vi "Dashboard Main.vi"() -> ()   [LabVIEW 2019]
uses:
  <vilib>/Utility/miscctls.llb/LVRowAndColumnTypeDef.ctl
  <vilib>/event_ctls.llb/eventvkey.ctl
  <vilib>/Rock Robotics/Network Tables/NT Read Numeric Array.vi
  <vilib>/Rock Robotics/WPI/Dashboard/WPI_DashboardLogging Global.vi
  <vilib>/Rock Robotics/Network Tables/NT Read Boolean.vi
panel:
  in  "Camera Settings Right":T1={"Frame Rate"=30, "Compression"=30, "Size"=1, "DB Camera Config"=FALSE} {"Frame Rate" scale=1.0..30.0; "Compression" scale=100.0..-1.0; "Size" items=["640x480", "320x240", "160x120"]}
  in  "Camera Name Right":string(combo)="No Camera Selection"
  out "Camera Perf":string
  in  "Camera Settings":T1={"Frame Rate"=30, "Compression"=30, "Size"=1, "DB Camera Config"=FALSE} {"Frame Rate" scale=1.0..30.0; "Compression" scale=100.0..-1.0; "Size" items=["640x480", "320x240", "160x120"]}
  in  "TCP":refnum<k5>
  in  "Rec Mode":enum32{"Stop", "Record", "Playback"}(radio)
  out "Robot IP":string
  out "Image Message":string="Timeout in Camera Communications"
  in  "Dashboard Tab":T2(tab)
  in  "Select Auto":string(combo)="Select Autonomous ..."
  out "NT Connection":bool
  out "MotorChart R":cluster{"Numeric":dbl, "Numeric":dbl}(graph)
  out "MotorChart L":cluster{"Numeric":dbl, "Numeric":dbl}(graph)
  out "MotorSliders R":cluster{"MotorSlide1":dbl, "MotorSlide2":dbl} {"MotorSlide2" scale=-1.0..1.0 scale format="%#_2e"; "MotorSlide1" scale=-1.0..1.0 scale format="%#_2e"}
  out "MotorSliders L":cluster{"MotorSlide1":dbl, "MotorSlide2":dbl} {"MotorSlide2" scale=-1.0..1.0 scale format="%#_2e"; "MotorSlide1" scale=-1.0..1.0 scale format="%#_2e"}
  out "Gyro":dbl(knob) scale=0.0..360.0
  out "JS1 Z":dbl(slide) scale=-1.0..1.0 scale format="%#_2e"
  out "JS1 Graph":cluster{"X":dbl, "Y":dbl}[](graph)
  out "JS1 Buttons":T3
  out "JS2 Z":dbl(slide) scale=-1.0..1.0 scale format="%#_2e"
  out "JS2 Graph":cluster{"X":dbl, "Y":dbl}[](graph)
  out "JS2 Buttons":T3
  out "Mode":T4(ring)=enum."Auto Disabled"
  out "Right Camera Perf":cluster{"Bandwidth (Mbps)":dbl, "FPS":dbl}
  out "x":sgl
  out "y":sgl
  out "Camera Image Right":T5(plugin-control)
  in  "DB/String 9":string
  in  "DB/String 8":string
  in  "DB/String 7":string
  in  "DB/String 6":string
  in  "DB/String 5":string
  in  "DB/String 4":string
  in  "DB/String 3":string
  in  "DB/String 2":string
  in  "DB/String 1":string
  in  "DB/String 0":string
  in  "DB/Slider 0":dbl(slide) scale=0.0..5.0
  in  "DB/Slider 1":dbl(slide) scale=0.0..5.0
  in  "DB/Slider 2":dbl(slide) scale=0.0..5.0
  in  "DB/Slider 3":dbl(slide) scale=0.0..5.0
  out "DB/LED 3":bool
  out "DB/LED 2":bool
  out "DB/LED 1":bool
  out "DB/LED 0":bool
  in  "DB/Button 3":bool
  in  "DB/Button 2":bool
  in  "DB/Button 1":bool
  in  "DB/Button 0":bool caption="New Name"
  in  "Test Slider":dbl(slide) scale=0.0..100.0 scale format="%#_3g"
  in  "On/Off":bool caption="Solenoid"
  in  "Test Name":u16(ring) items=["Select the test to run..."]
  in  "Test Tree":string(tree)
  in  "Motor":cluster{"Value":dbl, "Enable":bool} {"Value" scale=-1.0..1.0 scale format="%#_3g"}
  out "Progress":T6 {"Test Progress" scale=0.0..100.0}
  in  "Rev/Fwd":cluster{"Forward":bool, "Reverse":bool}
  in  "Test Ring":u16(ring) items=["Monochrome", "Color"]
  out "Cmd Status":string
  in  "Execute Command":bool
  in  "Command Params":string[][](table)
  in  "Command Selection":i32(listbox)
  in  "CheckList":i32(listbox)
  out "Tree":string(tree)
  out "Camera Image":T5(plugin-control)
  out "Background":bool
  in  "Camera Name":string(combo)="No Camera Selection"
  # "HW"
  # "HW"
  # "Joysticks"
  # "Drive Motors"
  # "Front"
  # "Right"
  # "Left"
  # "Back"
  # "This tab is a great place for autonomous settings and robot-specific values.\nPlace controls and indicators inside this tab and match name to\nDashboard Variables on robot. You can also delete this comment."
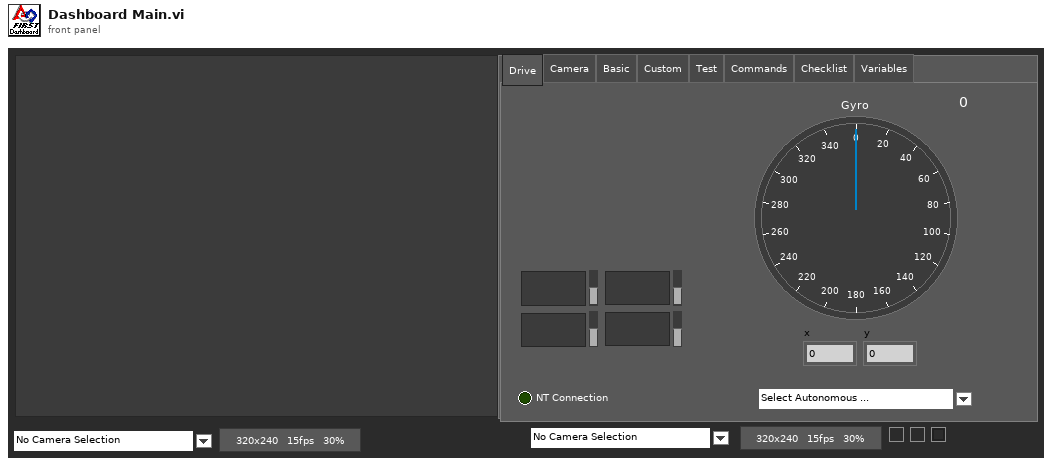
[diagram p1: front panel]
types:
  T1 = cluster{"Frame Rate":i32, "Compression":i32, "Size":u16, "DB Camera Config":bool}
  T2 = enum32{"Drive", "Camera", "Basic", "Custom", "Test", "Commands", "Checklist", "Variables"}
  T3 = cluster{bool, bool, bool, bool, bool, bool, bool, bool, bool, bool, bool, bool}
  T4 = enum8{"Tele-Op Disabled", "Tele-Op Enabled", "Auto Disabled", "Auto Enabled", "Test Disabled", "Test Enabled", "Disconnected", "No Code", "E-Stop"}
  T5 = typedef "IMAQ Image.ctl" = refnum<image>
  T6 = cluster{"Test Progress":u8, "Test Progress Text":string}
  T7 = cluster{"Save Path":path, "Interval (s)":dbl, "Keep":i32}
  T8 = typedef "Image Type" = u32
  T9 = cluster{"IDs":cluster{"RPC field ID":u16, "Unique ID":u16}, "String":string}
  T10 = cluster{"Camera Image":refnum<vi>, "Dashboard Tab":refnum<vi>, "Background":refnum<vi>, "Rec Mode":refnum<vi>, "Test Slider":refnum<vi>, "On/Off ":refnum<vi>, "Test Ring":refnum<vi>, "Rev/Fwd":refnum<vi>, "Test Name":refnum<vi>, "Motor":refnum<vi>, "Progress":refnum<vi>, "CheckList":refnum<vi>, "Tree":refnum<vi>, "Test Tree":refnum<vi>, "Command Params":refnum<vi>, "Command Selection":refnum<vi>, "Execute Command":refnum<vi>, "Cmd Status":refnum<vi>, "Camera Settings":refnum<vi>, "Camera Name":refnum<vi>, "Camera Perf":refnum<vi>, "Camera Settings Right":refnum<vi>, "Camera Name Right":refnum<vi>, "Camera Image Right":refnum<vi>}
  T11 = cluster{"Global Rectangle":i32[], "Contours":cluster{"Contour Type":u32, "ROI Type":u32, "Points":i32[]}[]}
  T12 = cluster{"Camera Name Right":string, string, "Saved DB Images Info":cluster{"Save Path":path, "Interval (s)":dbl, "Keep":i32}}
  T13 = cluster{"Error Strings":string, "Disable Counts":cluster{u16, u16}, "Rail Faults":cluster{u16, u16, u16}, "Robot IP":string, "DB Mode":u8, "Event Info":cluster{"Name":string, "Type":u8, "Number":u16, "Replay":u8}}
  T14 = cluster{"Storage":cluster{"Disk Free":u64, "RAM Block":u32, "RAM free":u32}, "CPU Utilization":cluster{"CPU % ISR":sgl, "CPU % Time Crit":sgl, "CPU % Timed Str":sgl, "CPU % High":sgl, "CPU % Above":sgl, "CPU % Normal":sgl, "CPU % Low":sgl}, "CAN":cluster{"% Bus Utilization":sgl, "Bus Off Cnt":u32, "TX_FIFO Full Cnt":u32, "Receive Error Cnt":u8, "Transmit Error Cnt":u8}, "HID":cluster{"HID Outputs":u32, "Rumble Low":u16, "Rumble High":u16}[]}
  T15 = cluster{"Status bits":cluster{"Test Mode":bool, "Autonomous":bool, "Enabled":bool, "Code Start":bool, "Brownout":bool, "Reserved 2":bool, "Reserved 3":bool, "E-Stop":bool}, "Code Trace":cluster{"Disabled":bool, "TeleOp":bool, "Auto":bool, "Test":bool}, "Controller Type":enum16{"unknown", "cRIO", "roboRio"}, "Code?":enum16{"unknown", "noCode", "code"}, "Battery V":dbl}
  T16 = cluster{"Control Bits":cluster{"TestMode":bool, "Autonomous":bool, "Enabled":bool, "FMS Present":bool, bool, bool, bool, "E-Stop":bool}, "Team Station ":u8, "Countdown":sgl, "Joystick Values":cluster{"Axes":dbl[], "Buttons":bool[], "POVs":i16[]}[]}
  T17 = cluster{"Axes":dbl[], "Buttons":bool[], "POVs":i16[]}[]
  T18 = cluster{"Axes":dbl[], "Buttons":bool[], "POVs":i16[]}
  T19 = cluster{"Buttons[0]":bool, "Buttons[1]":bool, "Buttons[2]":bool, "Buttons[3]":bool, "Buttons[4]":bool, "Buttons[5]":bool, "Buttons[6]":bool, "Buttons[7]":bool, "Buttons[8]":bool, "Buttons[9]":bool, "Buttons[10]":bool, "Buttons[11]":bool}
  T20 = cluster{"Camera Name":string, string, "Saved DB Images Info":cluster{"Save Path":path, "Interval (s)":dbl, "Keep":i32}}
  T21 = cluster{"Position":cluster{"x":sgl, "y":sgl}, "Angle":sgl, "Scale":sgl, "Score":sgl, "Bounding Box":cluster{"x":sgl, "y":sgl}[]}[]
  T22 = cluster{"Position":cluster{"x":sgl, "y":sgl}, "Angle":sgl, "Scale":sgl, "Score":sgl, "Bounding Box":cluster{"x":sgl, "y":sgl}[]}
  T23 = cluster{"Operation":enum16{"Update", "Clear"}, "Color Box":u32}[]
  T24 = typedef "eventvkey.ctl" = enum16{"ASCII", "Enter", "Return", "Shift", "Ctrl", "Alt", "Cmd", "Opt", "Caps", "NumLock", "Clear", "Break", "Up", "Down", "Left", "Right", "Insert", "Delete", "Home", "End", "PageUp", "PageDown", "Escape", "Help", "Pause", "ScrollLock", "F1", "F2", "F3", "F4", "F5", "F6", "F7", "F8", "F9", "F10", "F11", "F12", "F13", "F14", "F15", "F16", "F17", "F18", "F19", "F20", "F21", "F22", "F23", "F24", "Play", "VolumeUp", "VolumeDown", "Mute", "Two Byte Char"}
  T25 = cluster{"Image Size":bool, "Image Type":bool, "Pixel Value":bool, "ROI Information":bool, "Zoom Factor":bool}
  T26 = cluster{"Operation":enum16{"Update", "Clear"}, "Color Box":u32}
  T27 = typedef "LVRowAndColumnTypeDef.ctl" = cluster{"Row":i32, "Column":i32}
  T28 = cluster{"Shift":bool, "Ctrl":bool, "Alt":bool, "Cmd":bool, "Opt":bool}
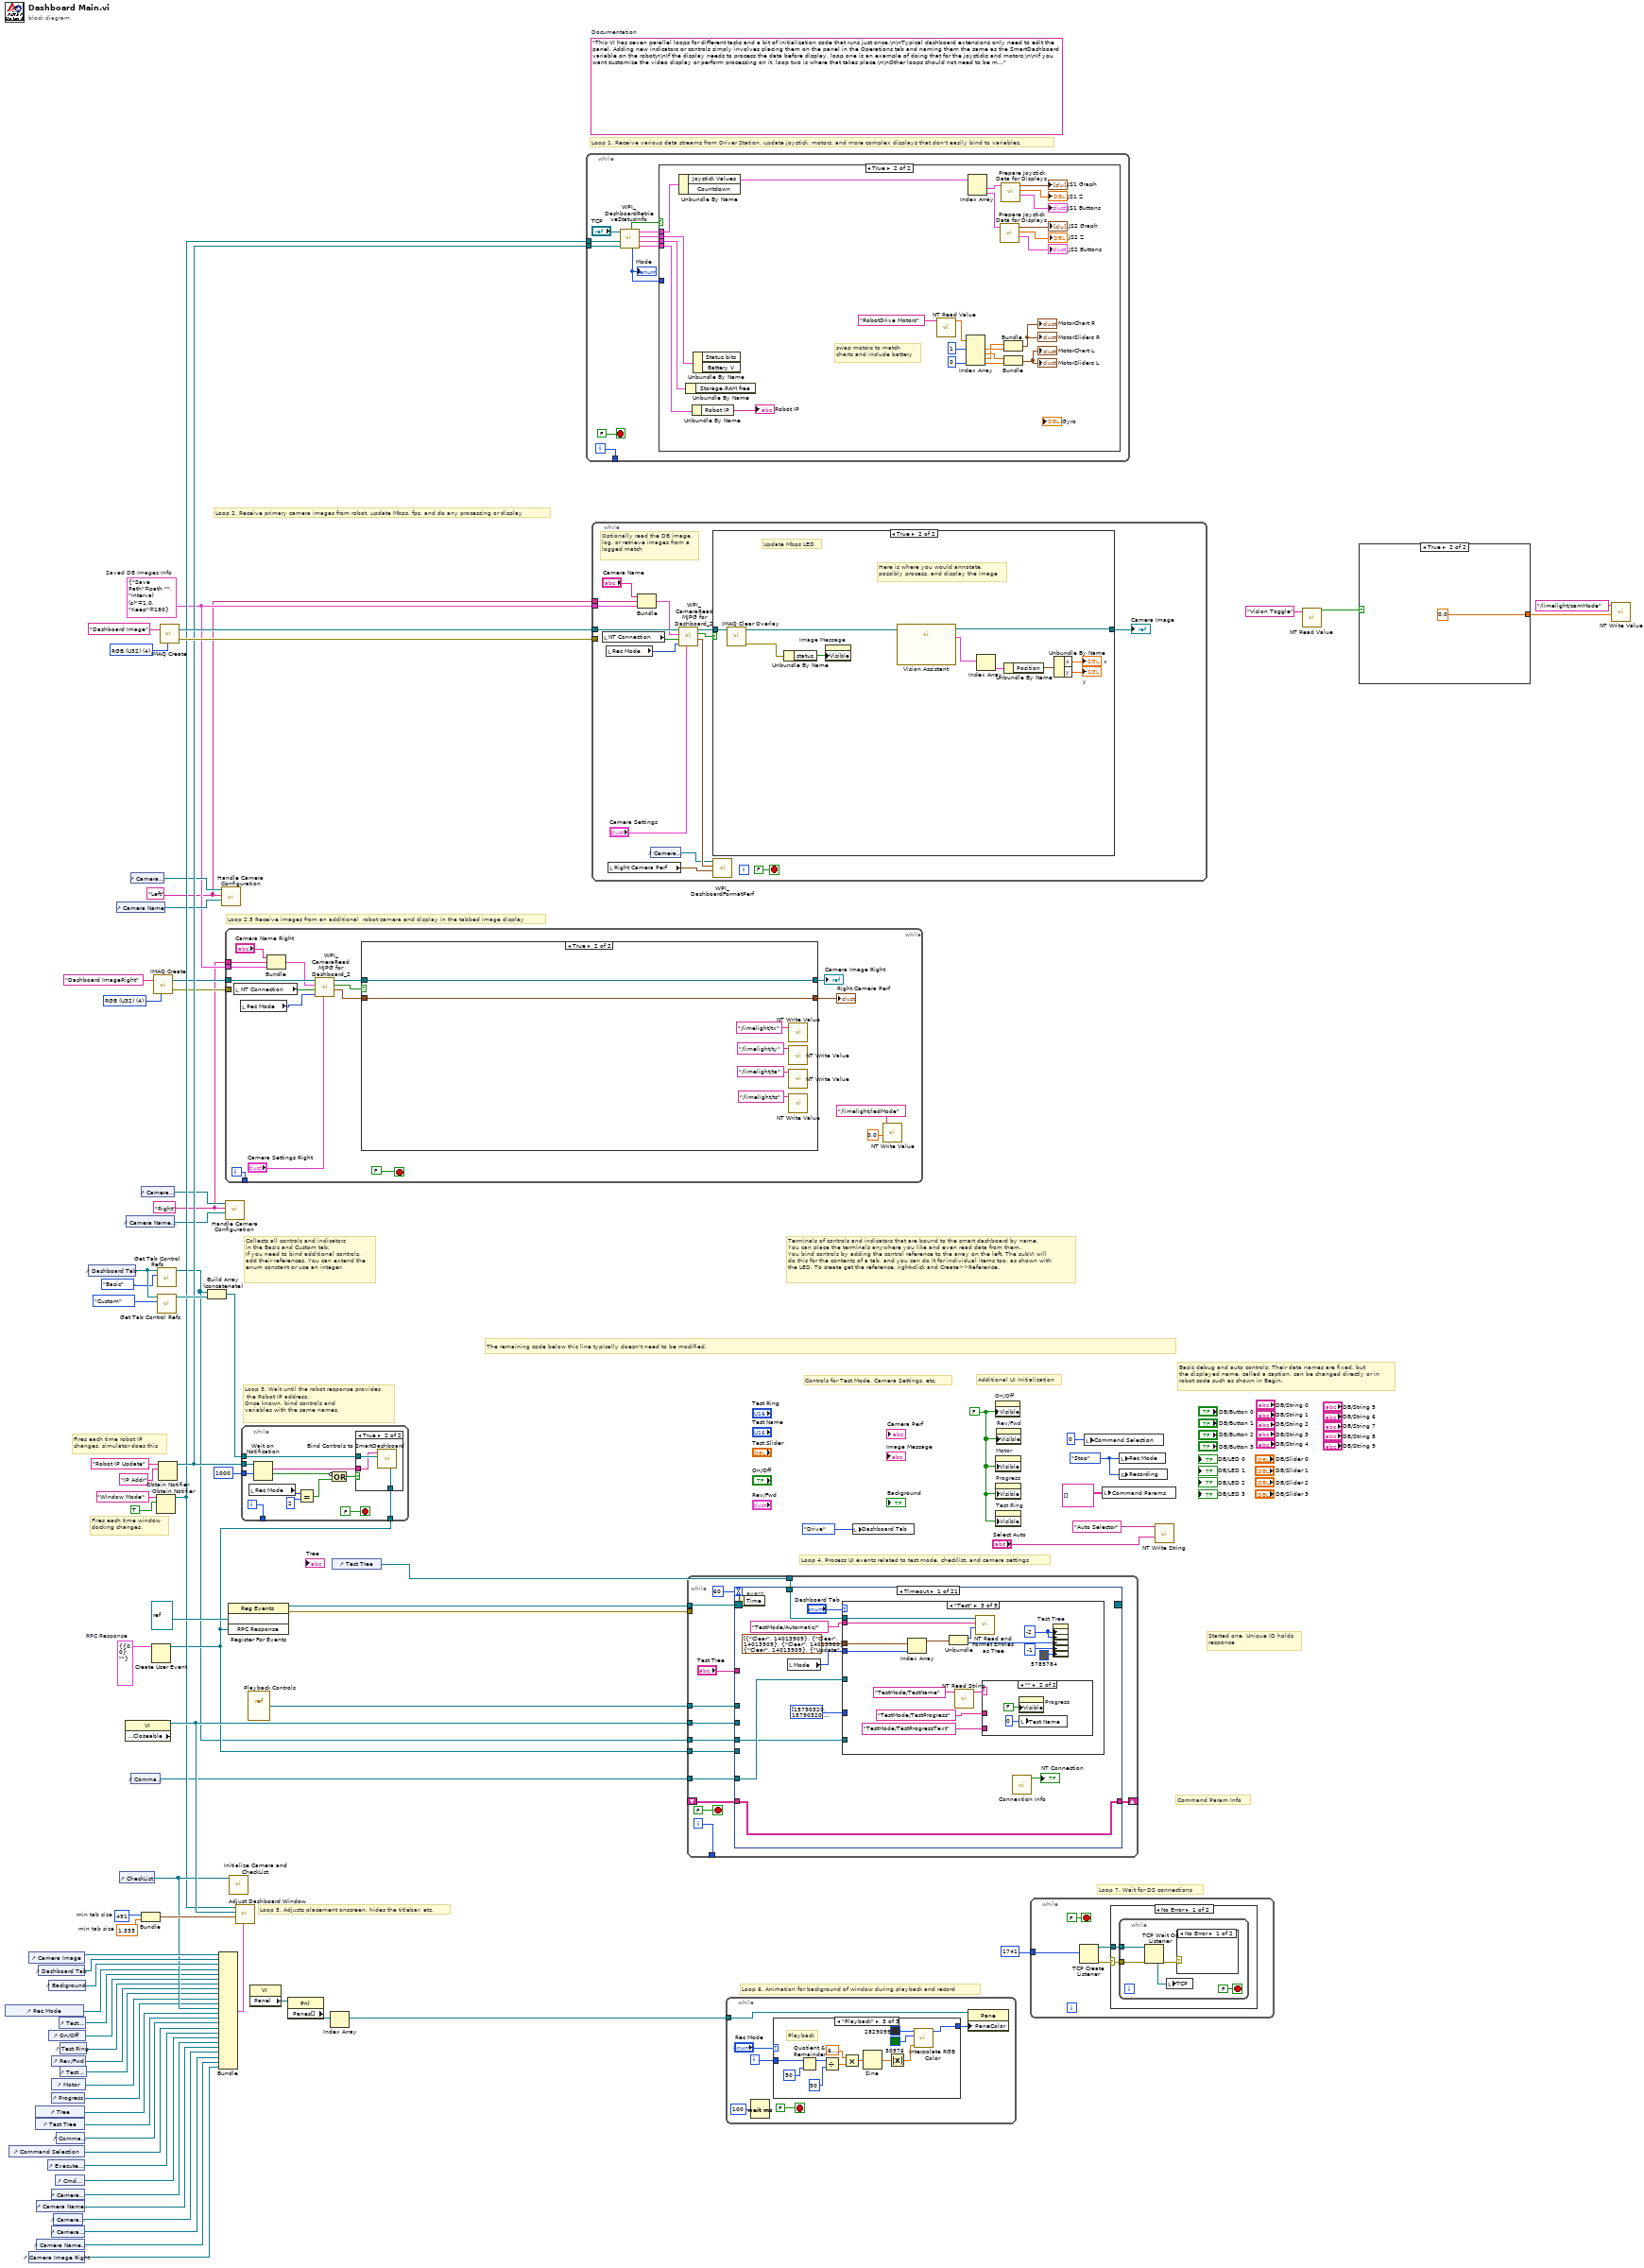
[diagram p0: block diagram]
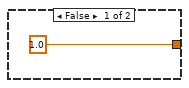
[diagram p2: hidden frame]
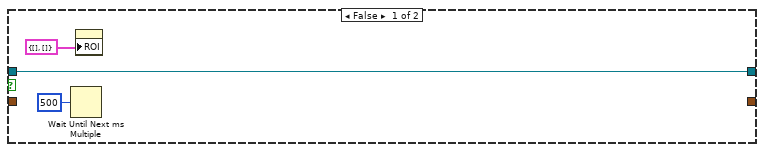
[diagram p3: hidden frame]
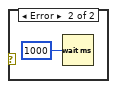
[diagram p4: hidden frame]
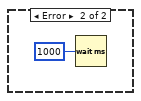
[diagram p5: hidden frame]
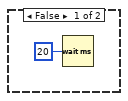
[diagram p6: hidden frame]
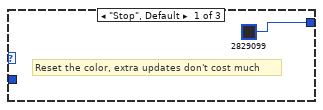
[diagram p7: hidden frame]
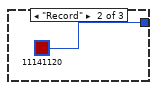
[diagram p8: hidden frame]
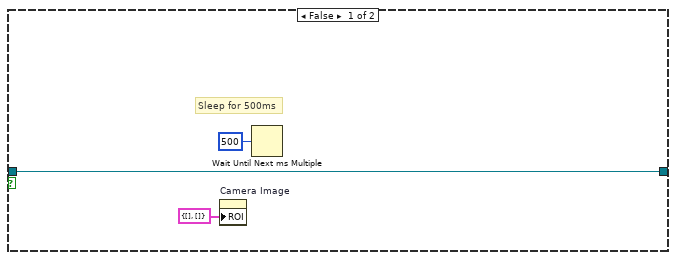
[diagram p10: hidden frame]
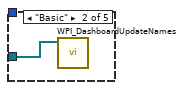
[diagram p12: hidden frame]
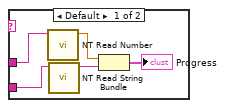
[diagram p13: hidden frame]
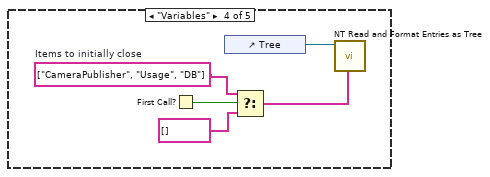
[diagram p14: hidden frame]
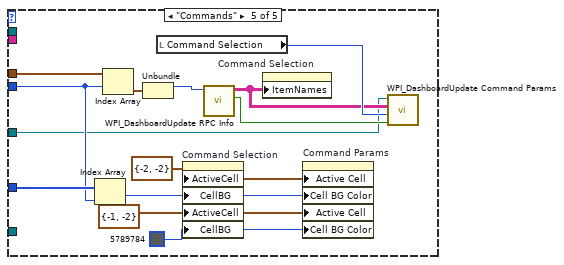
[diagram p15: hidden frame]
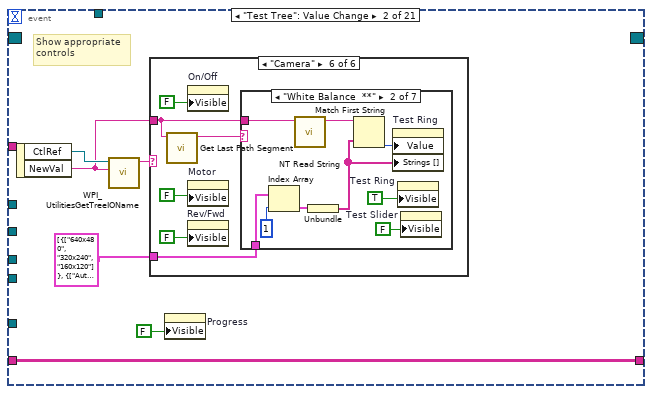
[diagram p16: hidden frame]
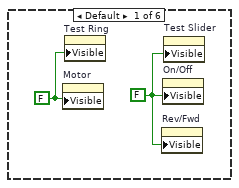
[diagram p17: hidden frame]
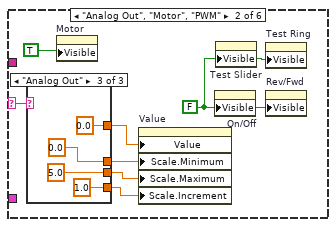
[diagram p18: hidden frame]
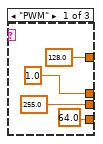
[diagram p19: hidden frame]
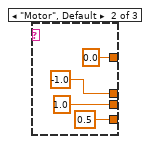
[diagram p20: hidden frame]
diagram:
  w7 = T7 {"Save Path"=path "", "Interval (s)"=1.0, "Keep"=180}  # Saved DB Images Info
  w6 = "Right"
  w5 = "Left"
  w17 = T8 4 items=["Grayscale (U8)", "Grayscale (I16)", "Grayscale (SGL)", "Complex (CSG)", "RGB (U32)", "HSL (U32)", "RGB (U64)"] ("Image Type")
  w33 = T9 {"IDs"={"RPC field ID"=0, "Unique ID"=0}, "String"=""}  # RPC Response
  w56 = 491  # min tab size
  w55 = 1.333  # min tab size
  w63 = enum32{"Stop", "Record", "Playback"}."Stop" ("Rec Mode")
  w40 = FALSE ("Visible")
  (unwired) "This VI has seven parallel loops for different tasks and a bit of initialization code that runs just once.\n\nTypical dashboard extensions only need to edit the panel. Adding new indicators or controls simply involves placing them on the panel in the Operations tab and naming them the same as the SmartDashboard variable on the robot\n\nIf the display needs to process the data before display, loop one is an example of doing that for the joysticks and motors.\n\nIf you want customize the video display or perform processing on it, loop two is where that takes place.\n\nOther loops should not need to be modified. They are pretty standard, and document the task they perform."  # Documentation
  w80 = T8 4 items=["Grayscale (U8)", "Grayscale (I16)", "Grayscale (SGL)", "Complex (CSG)", "RGB (U32)", "HSL (U32)", "RGB (U64)"] ("Image Type")
  # "Loop 2.5 Receive images from an additional  robot camera and display in the tabbed image display"
  # "Command Param Info"
  # "Started one, Unique ID holds\nresponse"
  # "Loop 7. Wait for DS connections"
  # "Basic debug and auto controls: Their data names are fixed, but\nthe displayed name, called a caption, can be changed directly or in\nrobot code such as shown in Begin."
  # "Controls for Test Mode, Camera Settings, etc."
  # "Additional UI Initialization"
  # "Loop 6. Animation for background of window during playback and record"
  # "Fires each time robot IP\nchanges, simulator does this"
  # "Fires each time window\ndocking changes."
  # "Collects all controls and indicators\nin the Basic and Custom tab.\nIf you need to bind additional controls,\nadd their references. You can extend the\nenum constant or use an integer."
  # "The remaining code below this line typically doesn't need to be modified."
  # "Loop 4. Process UI events related to test mode, checklist, and camera settings"
  # "Terminals of controls and indicators that are bound to the smart dashboard by name.\nYou can place the terminals anywhere you like and even read data from them.\nYou bind controls by adding the control reference to the array on the left. The subVI will\ndo this for the contents of a tab, and you can do it for individual items too, as shown with\nthe LED. To create get the reference, right-click and Create>>Reference."
  # "Loop 3. Wait until the robot response provides\n the Robot IP address.\nOnce known, bind controls and\nvariables with the same names."
  # "Loop 5. Adjusts placement onscreen, hides the titlebar, etc."
  # "Loop 1. Receive various data streams from Driver Station, update joystick, motors, and more complex displays that don't easily bind to variables."
  # "Loop 2. Receive primary camera images from robot, update Mbps, fps, and do any processing or display"
  n1 = control-ref of="Rec Mode"() -> (w46:refnum<vi>)
  n2 = control-ref of="Command Selection"() -> (w32:refnum<vi>)
  n3 = control-ref of="Camera Image Right"() -> (w10:refnum<vi>)
  n4 = control-ref of="Camera Image"() -> (w58:refnum<vi>)
  n5 = control-ref of="Tree"() -> (w50:refnum<vi>)
  n6 = control-ref of="Test Tree"() -> (w49:refnum<vi>)
  n7 = control-ref of="Camera Name"() -> (w23:refnum<vi>)
  n8 = control-ref of="Camera Name Right"() -> (w11:refnum<vi>)
  n9 = control-ref of="Dashboard Tab"() -> (w57:refnum<vi>)
  n10 = control-ref of="Execute Command"() -> (w34:refnum<vi>)
  n11 = control-ref of="Background"() -> (w53:refnum<vi>)
  n12 = control-ref of="On/Off"() -> (w44:refnum<vi>)
  n13 = control-ref of="Progress"() -> (w41:refnum<vi>)
  n14 = control-ref of="Camera Settings"() -> (w24:refnum<vi>)
  n15 = control-ref of="Camera Settings Right"() -> (w12:refnum<vi>)
  n16 = control-ref of="Rev/Fwd"() -> (w42:refnum<vi>)
  n17 = control-ref of="Motor"() -> (w47:refnum<vi>)
  n18 = control-ref of="Camera Perf"() -> (w22:refnum<vi>)
  n19 = control-ref of="Cmd Status"() -> (w28:refnum<vi>)
  n20 = control-ref of="Command Params"() -> (w35:refnum<vi>)
  n21 = control-ref of="Test Slider"() -> (w45:refnum<vi>)
  n22 = control-ref of="Test Ring"() -> (w43:refnum<vi>)
  n23 = control-ref of="Test Name"() -> (w48:refnum<vi>)
  n24 = control-ref of="Dashboard Tab"() -> (w61:refnum<vi>)
  n25 = control-ref of="Camera Name"() -> (w25:refnum<vi>)
  n26 = control-ref of="CheckList"() -> (w51:refnum<vi>)
  n27 = property class="VI" props=["Front Panel.Closeable"]() -> (reference out=w62:refnum<vi>)  [unwired: 2 in, 2 out]
  n28 = control-ref of="Camera Name Right"() -> (w13:refnum<vi>)
  n29 = control-ref of="Camera Settings"() -> (w26:refnum<vi>)
  n30 = control-ref of="Command Params"() -> (w27:refnum<vi>)
  n31 = control-ref of="Camera Settings Right"() -> (w14:refnum<vi>)
  n32 = Bundle("min tab size"=w56, "min tab size"=w55) -> (w54:cluster{"min tab size":i32, "min tab size":dbl})  [unwired: 1 in]
  n33 = Create User Event(user event datatype=w33) -> (user event=w29:refnum<user-event>)  [unwired: 1 in, 1 out]
  n34 = call "IMAQ Create"("Image Name"="Dashboard ImageRight", "Image Type"=w17) -> ("New Image"=w16:T5, "error out"=w15:errorcluster)  [unwired: 2 in, 1 out]
  n35 = Obtain Notifier(name (unnamed)="Window Mode", notification data type=TRUE) -> (notifier out=w38:refnum<notifier>)  [unwired: 2 in, 2 out]
  n36 = call <vilib>:"Get Tab Control Refs.vi"("Page Index"=T2."Basic" ("Dashboard Tab"), "TabControl in"=w61) -> ("ControlsOnPage"=w21:refnum<vi>[])  [unwired: 9 in]
  n37 = call <vilib>:"Get Tab Control Refs.vi"("Page Index"=T2."Custom" ("Dashboard Tab"), "TabControl in"=w61) -> ("ControlsOnPage"=w60:refnum<vi>[])  [unwired: 9 in]
  n38 = Obtain Notifier(name (unnamed)="Robot IP Update", notification data type="IP Addr" ("name (unnamed)")) -> (notifier out=w39:refnum<notifier>)  [unwired: 2 in, 2 out]
  n39 = call "IMAQ Create"("Image Name"="Dashboard Image", "Image Type"=w80) -> ("New Image"=w78:T5, "error out"=w77:errorcluster)  [unwired: 2 in, 1 out]
  n40 = Build Array (concatenate)(w21, w60) -> (w59:refnum<vi>[])
  n41 = Bundle("Camera Image"=w58, "Dashboard Tab"=w57, "Background"=w53, "Rec Mode"=w46, "Test Slider"=w45, "On/Off"=w44, "Test Ring"=w43, "Rev/Fwd"=w42, "Test Name"=w48, "Motor"=w47, "Progress"=w41, "CheckList"=w51, "Tree"=w50, "Test Tree"=w49, "Command Params"=w35, "Command Selection"=w32, "Execute Command"=w34, "Cmd Status"=w28, "Camera Settings"=w24, "Camera Name"=w23, "Camera Perf"=w22, "Camera Settings Right"=w12, "Camera Name Right"=w11, "Camera Image Right"=w10) -> (w52:T10)  [unwired: 1 in]
  n42 = call "Handle Camera Configuration.vi"("CameraNameRef"=w25, "Display Name"=w5, "ClusterRef"=w26) -> ()  [unwired: 9 in]
  n43 = call "Handle Camera Configuration.vi"("CameraNameRef"=w13, "Display Name"=w6, "ClusterRef"=w14) -> ()  [unwired: 9 in]
  n44 = while {
    tunnel: w16 -> [w97]
    tunnel: w15 -> [_]
    tunnel: [w92] -> _
    tunnel: w7 -> [w89]
    tunnel: w6 -> [w86]
    i -> [w92]
    stop <- FALSE stop-if-true
    n45 = local read "NT Connection"() -> (w90:bool)
    n46 = local read "Rec Mode"() -> (w96:enum32{"Stop", "Record", "Playback"})
    n47 = Bundle("Camera Name Right"="Camera Name Right", w86, "Saved DB Images Info"=w89) -> (w88:T12)  [unwired: 1 in]
    n48 = call <vilib>:"WPI_CameraRead MJPG for Dashboard_2.vi"("Camera Settings"="Camera Settings Right", "Rec Mode"=w96, "NT Connection"=w90, "Capture Info"=w88, "Image in"=w97) -> ("perf info"=w84:cluster{"Bandwidth (Mbps)":dbl, "fps":dbl}, "Active"=w91:bool, "Image\\ out"=w94:T5)  [unwired: 4 in]
    n49 = case shown="True" w91 {
      tunnel: w94 -> [w99 w101]
      tunnel: [w99 w101] -> w81
      tunnel: [_ w106] -> w85
      tunnel: w84 -> [_ w106]
      frame False {
        n50 = Wait Until Next ms Multiple(millisecond multiple=u32 500) -> ()  [unwired: 1 out]
        n51 = property on="Camera Image Right" class="ImageControl"("ROI"=T11 {"Global Rectangle"=[], "Contours"=[]}) -> ()  [unwired: 2 in, 2 out]
      }
      frame True {
        n52 = call-poly <vilib>:"NT Write Value.vi"("Name"="/limelight/tx") -> ()  [unwired: 10 in, 1 out]
        n53 = call-poly <vilib>:"NT Write Value.vi"("Name"="/limelight/ty") -> ()  [unwired: 10 in, 1 out]
        n54 = call-poly <vilib>:"NT Write Value.vi"("Name"="/limelight/ta") -> ()  [unwired: 10 in, 1 out]
        n55 = call-poly <vilib>:"NT Write Value.vi"("Name"="/limelight/ts") -> ()  [unwired: 10 in, 1 out]
      }
    }
    "Right Camera Perf" <- w85
    "Camera Image Right" <- w81
    n56 = call-poly <vilib>:"NT Write Value.vi"("Numeric"=0.0, "Name"="/limelight/ledMode") -> ()  [unwired: 9 in, 1 out]
  }
  n57 = register-events(refnum<vi> refnum, w29) -> (reference out=w67:refnum<event-registration>, error out=w66:errorcluster)  [unwired: 2 in]
  n58 = call "Initialize Camera and CheckList.vi"("ListBox in"=w51) -> ()  [unwired: 11 in]
  n59 = call "Adjust Dashboard Window.vi"("Sizing Refnums"=w52, "Size Constraints"=w54, "VI"=w62, "WIn Mode"=w38) -> ()  [unwired: 8 in]
  n60 = while {
    tunnel: w59 -> [w118]
    tunnel: w39 -> [w116]
    tunnel: [w114] -> _
    tunnel: u32 1000 ("milliseconds to wait") -> [w113]
    tunnel: w29 -> [w107]
    i -> [w114]
    stop <- FALSE stop-if-true
    n61 = local read "Rec Mode"() -> (w109:enum32{"Stop", "Record", "Playback"})
    n62 = Wait on Notification(notifier=w116, timeout in ms (-1)=w113) -> (notification=w115:string, timed out?=w111:bool)  [unwired: 2 in, 2 out]
    n63 = Equal?(x=w109, y=u16 2 ("Rec Mode")) -> (x = y?=w110:bool)
    n64 = Compound Arithmetic op=OR(invert w111, w110) -> (w112:bool)
    n65 = case shown="True" w112 {
      tunnel: w118 -> [_ w121]
      tunnel: w115 -> [_ w120]
      tunnel: w107 -> [_ w119]
      frame False {
      }
      frame True {
        n66 = call <vilib>:"Bind Controls to SmartDashboard.vi"("RPC ref"=w119, "Bound Control Refs"=w121, "Server IP Address"=w120) -> ()  [unwired: 9 in]
      }
    }
  }
  n67 = vi-ref "Playback Controls.vi"() -> (w68:refnum<vi>)
  n68 = property class="VI"() -> ("Panel"=w70:refnum<vi>)  [unwired: 2 in, 2 out]
  n69 = property class="Pnl"(reference=w70) -> ("Panes[]"=w71:refnum<vi>[])  [unwired: 1 in, 2 out]
  n70 = Index Array(array=w71) -> (element=w69:refnum<vi>)  [unwired: 1 in]
  n71 = control-ref of="Test Tree"() -> (w72:refnum<vi>)
  n72 = while {
    tunnel: [w131] -> _
    tunnel: w39 -> [w125]
    tunnel: w38 -> [w122]
    i -> [w131]
    stop <- FALSE stop-if-true
    n73 = call <vilib>:"WPI_DashboardRetrieveStatusInfo.vi"("Binding Refnum"=w125, "Window Mode Notifier"=w122, "TCP Cnx"="TCP") -> ("Power and Errors"=w126:T13, "Robot Metrics"=w129:T14, "Status Info"=w130:T15, "Control Info"=w127:T16, "Robot Mode"=w124:T4, "Process?"=w128:bool)  [unwired: 3 in]
    "Mode" <- w124
    n74 = case shown="True" w128 {
      tunnel: w130 -> [_ w157]
      tunnel: w129 -> [_ w156]
      tunnel: w127 -> [_ w155]
      tunnel: w126 -> [_ w154]
      tunnel: w124 -> [_ _]
      frame False {
        n75 = Wait (ms)(milliseconds to wait=u32 20) -> ()  [unwired: 1 out]
      }
      frame True {
        # "swap motors to match\ncharts and include battery"
        n76 = Unbundle By Name(w155) -> ("Joystick Values"=w145:T17)  [unwired: 1 out]
        n77 = Unbundle By Name(w156) -> ()  [unwired: 1 out]
        n78 = Unbundle By Name(w154) -> ("Robot IP"=→"Robot IP":string)
        n79 = Unbundle By Name(w157) -> ()  [unwired: 2 out]
        n80 = call-poly <vilib>:"NT Read Value.vi"("Name"="RobotDrive Motors") -> ("Numeric Array"=w135:dbl[])  [unwired: 9 in, 1 out]
        n81 = Index Array(array=w135, index #1=1, index #4=0) -> (element #1=w149:dbl, element #2=w150:dbl, element #3=w148:dbl, element #4=w153:dbl)  [unwired: 2 in]
        n82 = Index Array(array=w145) -> (element #1=w144:T18, element #2=w140:T18)  [unwired: 2 in]
        n83 = call "Prepare Joystick Data for Displays.vi"("Joystick Values"=w140) -> ("Buttons"=→"JS2 Buttons":T19, "Z Axis"=→"JS2 Z":dbl, "Cartesian Data"=→"JS2 Graph":cluster{"X axis":dbl, "X axis":dbl}[])  [unwired: 8 in]
        n84 = call "Prepare Joystick Data for Displays.vi"("Joystick Values"=w144) -> ("Buttons"=→"JS1 Buttons":T19, "Z Axis"=→"JS1 Z":dbl, "Cartesian Data"=→"JS1 Graph":cluster{"X axis":dbl, "X axis":dbl}[])  [unwired: 8 in]
        n85 = Bundle("Numeric"=w148, "Numeric"=w149) -> (→"MotorChart R" →"MotorSliders R":cluster{"Numeric":dbl, "Numeric":dbl})  [unwired: 1 in]
        n86 = Bundle("Numeric"=w150, "Numeric"=w153) -> (→"MotorChart L" →"MotorSliders L":cluster{"Numeric":dbl, "Numeric":dbl})  [unwired: 1 in]
      }
    }
  }
  n87 = while {
    tunnel: w78 -> [w171]
    tunnel: w77 -> [_]
    tunnel: w7 -> [w165]
    tunnel: w5 -> [w162]
    stop <- FALSE stop-if-true
    # "Optionally read the DB image,\nlog, or retrieve images from a\nlogged match"
    n88 = local read "NT Connection"() -> (w166:bool)
    n89 = local read "Rec Mode"() -> (w168:enum32{"Stop", "Record", "Playback"})
    n90 = local read "Right Camera Perf"() -> (w160:cluster{"Bandwidth (Mbps)":dbl, "FPS":dbl})
    n91 = Bundle("Camera Name"="Camera Name", w162, "Saved DB Images Info"=w165) -> (w164:T20)  [unwired: 1 in]
    n92 = control-ref of="Camera Perf"() -> (w159:refnum<vi>)
    n93 = call <vilib>:"WPI_CameraRead MJPG for Dashboard_2.vi"("Camera Settings"="Camera Settings", "Rec Mode"=w168, "NT Connection"=w166, "Capture Info"=w164, "Image in"=w171) -> ("perf info"=w161:cluster{"Bandwidth (Mbps)":dbl, "fps":dbl}, "Active"=w169:bool, "Image\\ out"=w170:T5)  [unwired: 4 in]
    n94 = case shown="True" w169 {
      tunnel: w170 -> [w174 w183]
      tunnel: [w174 w181] -> w158
      frame False {
        # "Sleep for 500ms"
        n95 = property on="Camera Image" class="ImageControl"("ROI"=T11 {"Global Rectangle"=[], "Contours"=[]}) -> ()  [unwired: 2 in, 2 out]
        n96 = Wait Until Next ms Multiple(millisecond multiple=u32 500) -> ()  [unwired: 1 out]
      }
      frame True {
        # "Here is where you would annotate,\npossibly process, and display the image"
        # "Update Mbps LED"
        n97 = call "IMAQ Clear Overlay"("Image"=w183) -> ("error out"=w184:errorcluster, "Image Out"=w182:T5)  [unwired: 2 in, 7 out]
        n98 = Unbundle By Name(w184) -> ("status"=w185:bool)
        n99 = property on="Image Message" class="Str"("Visible"=w185) -> ()  [unwired: 2 in, 2 out]
        n100 = call "Vision Assistant"("Image In"=w182) -> ("Image Out"=w181:T5, "Matches (Pattern Matching 1)"=w180:T21)  [unwired: 24 in, 1 out]
        n101 = Index Array(array=w180) -> (element=w179:T22)  [unwired: 1 in]
        n102 = Unbundle By Name(w179) -> ("Position"=w178:cluster{"x":sgl, "y":sgl})
        n103 = Unbundle By Name(w178) -> ("x"=→"x":sgl, "y"=→"y":sgl)
      }
    }
    "Camera Image" <- w158
    n104 = call <vilib>:"WPI_DashboardFormatPerf.vi"("Right Camera Perf"=w160, "Performance"=w161, "String in"=w159) -> ()  [unwired: 9 in]
  }
  n105 = while {
    tunnel: [w195] -> _
    tunnel: w72 -> [w194]
    tunnel: w68 -> [w193]
    tunnel: w67 -> [w192]
    tunnel: w66 -> [_]
    tunnel: w62 -> [w191]
    tunnel: w29 -> [w190]
    tunnel: w27 -> [w189]
    shift-right: [w188] -> _
    shift-left: _ -> [w187]
    tunnel: w21 -> [w186]
    i -> [w195]
    stop <- FALSE stop-if-true
    n106 = event shown="[0] Timeout" {
      selector: w192 -> [_ _ _ _ _ _ _ _ _ _ _ _ _ _ _ _ _ _ _ _ _]
      dyn-events: [_ _ _ _ _ _ _ _ _ _ _ _ _ _ _ _ w455 _ _ _ _] -> _
      timeout: u32 60 ("milliseconds to wait") -> [_ _ _ _ _ _ _ _ _ _ _ _ _ _ _ _ _ _ _ _ _]
      tunnel: w194 -> [w207 _ _ _ _ _ _ _ _ _ _ _ _ _ _ _ _ _ _ _ _]
      tunnel: "Test Tree" -> [_ _ _ _ _ _ _ _ _ _ _ w422 w430 w432 w436 w444 _ _ _ _ _]
      tunnel: w193 -> [_ _ _ _ _ _ _ _ _ _ _ _ _ _ _ _ w457 _ w475 _ _]
      tunnel: w191 -> [_ _ _ _ _ _ _ _ _ _ _ _ _ _ _ _ w453 _ _ _ _]
      tunnel: w190 -> [_ _ _ _ _ _ _ _ _ _ _ _ _ _ _ _ w451 _ _ _ _]
      tunnel: w189 -> [w202 _ _ _ _ _ w373 _ _ _ _ _ _ _ _ _ _ _ _ _ _]
      tunnel: [w201 w250 w352 w357 w366 w370 w371 w380 w390 w397 w409 w421 w428 w431 w435 w443 w450 w470 w472 w476 w489] -> w188
      tunnel: w187 -> [w201 w250 w352 w357 w366 w370 w371 _ _ w397 w409 w421 w428 w431 w435 w443 w450 w470 w472 w476 w489]
      tunnel: w186 -> [w199 _ _ _ _ _ _ _ _ _ _ _ _ _ _ _ _ _ _ _ _]
      event Timeout {
        n107 = event-data() -> ()  [unwired: 1 in, 1 out]
        n108 = local read "Mode"() -> (w204:T4)
        n109 = case shown="\"Test\"" "Dashboard Tab" {
          tunnel: w207 -> [_ _ w223 _ _]
          tunnel: "TestMode/Automatic/" ("Name Pattern") -> [_ _ w222 _ _]
          tunnel: T23 [{"Operation"=enum."Clear", "Color Box"=14013909}, {"Operation"=enum."Clear", "Color Box"=14013909}, {"Operation"=enum."Clear", "Color Box"=14013909}, {"Operation"=enum."Clear", "Color Box"=14013909}, {"Operation"=enum."Update", "Color Box"=14013909}, {"Operation"=enum."Update", "Color Box"=16777215}, {"Operation"=enum."Clear", "Color Box"=14013909}, {"Operation"=enum."Clear", "Color Box"=14013909}, {"Operation"=enum."Clear", "Color Box"=14013909}] -> [_ _ w215 _ w243]
          tunnel: w204 -> [_ _ w214 _ w242]
          tunnel: u32[] [15790320, 15790320, 15790320, 15790320, 16777215, 16777215, 15790320, 15790320, 15790320] -> [_ _ _ _ w248]
          tunnel: w202 -> [_ _ _ _ w236]
          tunnel: w199 -> [_ w209 _ _ _]
          frame "Custom", Default {
          }
          frame "Basic" {
            n110 = call <vilib>:"WPI_DashboardUpdateNames.vi"("Controls on Tab"=w209) -> ()  [unwired: 11 in]
          }
          frame "Test" {
            w221 = -2 ("Active Item:Row Number")
            n111 = Index Array(array=w215, index=w214) -> (element=w216:T26)
            n112 = Unbundle(w216) -> ("Operation"=w217:enum16{"Update", "Clear"}, "Color Box"=w218:u32)
            n113 = call <vilib>:"NT Read String.vi"("Name"="TestMode/TestName") -> ("String"=w212:string)  [unwired: 9 in, 1 out]
            n114 = call <vilib>:"NT Read and Format Entries as Tree.vi"("Operation"=w217, "Name Pattern"=w222, "Tree Refnum"=w223) -> ()  [unwired: 7 in, 2 out]
            n115 = case shown="\"\"" w212 {
              tunnel: "TestMode/TestProgress" ("Name") -> [w225 _]
              tunnel: "TestMode/TestProgressText" ("Name") -> [w224 _]
              frame Default {
                n116 = call <vilib>:"NT Read Number.vi"("Name"=w225) -> ("Numeric"=w226:dbl)  [unwired: 9 in, 1 out]
                n117 = call <vilib>:"NT Read String.vi"("Name"=w224) -> ("String"=w227:string)  [unwired: 9 in, 1 out]
                n118 = Bundle("Numeric"=w226, "String"=w227) -> (→"Progress":cluster{"Numeric":dbl, "String":string})  [unwired: 1 in]
              }
              frame "" {
                n119 = property on="Progress" class="Clust (strict)"("Visible"=FALSE) -> ()  [unwired: 2 in, 2 out]
                n120 = local write "Test Name"(u16 0) -> ()
              }
            }
            n121 = property on="Test Tree" class="Tree (strict)"("Active Item Row Number"=w221, "ActiveColNum"=w221, "CellBG"=w218, "Active Item Row Number"=-1 ("Active Item:Row Number"), "CellBG"=u32 5789784 ("Color Box")) -> ()  [unwired: 2 in, 2 out]
          }
          frame "Variables" {
            w233 = string[] ["CameraPublisher", "Usage", "DB"]  # Items to initially close
            n122 = First Call?() -> (First Call?: T/F=w234:bool)
            n123 = control-ref of="Tree"() -> (w235:refnum<vi>)
            n124 = Select(t=w233, s=w234, f=string[] []) -> (s? t:f=w231:string[])
            n125 = call <vilib>:"NT Read and Format Entries as Tree.vi"("Tags to  Close"=w231, "Tree Refnum"=w235) -> ()  [unwired: 8 in, 2 out]
          }
          frame "Commands" {
            w244 = u32 5789784 ("Color Box")
            w245 = T27 {"Row"=-1, "Column"=-2} ("Active Cell:Active Cell")
            w247 = T27 {"Row"=-2, "Column"=-2} ("Active Cell:Active Cell")
            n126 = Index Array(array=w248, index=w242) -> (element=w246:u32)
            n127 = Index Array(array=w243, index=w242) -> (element=w241:T26)
            n128 = Unbundle(w241) -> ("Operation"=w240:enum16{"Update", "Clear"})  [unwired: 1 out]
            n129 = local read "Command Selection"() -> (w239:i32)
            n130 = property on="Command Selection" class="MCListbox (strict)"("ActiveCell"=w247, "CellBG"=w246, "ActiveCell"=w245, "CellBG"=w244) -> ()  [unwired: 2 in, 2 out]
            n131 = call <vilib>:"WPI_DashboardUpdate RPC Info.vi"("Operation"=w240) -> ("update"=w238:bool, "commands"=w237:string[][])  [unwired: 9 in]
            n132 = property on="Command Selection" class="MCListbox (strict)"("ItemNames"=w237) -> ()  [unwired: 2 in, 2 out]
            n133 = property on="Command Params" class="Tbl (strict)"("Active Cell"=w247, "Cell BG Color"=w246, "Active Cell"=w245, "Cell BG Color"=w244) -> ()  [unwired: 2 in, 2 out]
            n134 = call <vilib>:"WPI_DashboardUpdate Command Params.vi"("Update"=w238, "NewVal"=w239, "Commands"=w237, "Param Tbl"=w236) -> ()  [unwired: 7 in, 1 out]
          }
        }
        n135 = call <vilib>:"Connextion Info.vi"() -> ("Connected"=→"NT Connection":bool)  [unwired: 10 in, 1 out]
      }
      event "Test Tree": Value Change {
        # "Show appropriate\ncontrols"
        n136 = event-data() -> ("CtlRef"=w253:refnum<vi>, "NewVal"=w251:string)  [unwired: 1 in]
        n137 = call <vilib>:"WPI_UtilitiesGetTreeIOName.vi"("NewVal"=w251, "TreeControl in"=w253) -> ("I/O Name"=w254:string)  [unwired: 9 in]
        n138 = case shown="\"Camera\"" w254 {
          selector: w254 -> [_ w261 _ w283 w292 _]
          tunnel: w251 -> [_ _ w280 w282 _ w299]
          tunnel: cluster{string[]}[] [{["640x480", "320x240", "160x120"]}, {["Auto", "Fixed indoor", "Fixed outdoor 1", "Fixed outdoor 2", "Fixed fluorescent 1", "Fixed fluorescent 2", "Hold current"]}, {["Auto", "Flicker-free 50 Hz", "Flicker-free 60 Hz", "Hold current"]}, {["None", "Prioritize frame rate", "Prioritize image quality"]}, {["Monochrome", "Color"]}] -> [_ _ _ _ _ w298]
          frame Default {
            w256 = FALSE ("Visible")
            w255 = FALSE ("Visible")
            n139 = property on="Motor" class="Clust (strict)"("Visible"=w255) -> ()  [unwired: 2 in, 2 out]
            n140 = property on="Test Ring" class="Ring (strict)"("Visible"=w255) -> ()  [unwired: 2 in, 2 out]
            n141 = property on="Rev/Fwd" class="Clust (strict)"("Visible"=w256) -> ()  [unwired: 2 in, 2 out]
            n142 = property on="On/Off" class="Bool (strict)"("Visible"=w256) -> ()  [unwired: 2 in, 2 out]
            n143 = property on="Test Slider" class="Slide (strict)"("Visible"=w256) -> ()  [unwired: 2 in, 2 out]
          }
          frame "Analog Out", "Motor", "PWM" {
            w262 = FALSE ("Visible")
            n144 = case shown="\"Analog Out\"" w261 {
              tunnel: [1.0 ("Value") -1.0 ("Value") 0.0 ("Value")] -> w260
              tunnel: [255.0 ("Value") 1.0 ("Value") 5.0 ("Value")] -> w259
              tunnel: [128.0 ("Value") 0.0 ("Value") 0.0 ("Value")] -> w258
              tunnel: [64.0 ("Value") 0.5 ("Value") 1.0 ("Value")] -> w257
              frame "PWM" {
              }
              frame "Motor", Default {
              }
              frame "Analog Out" {
              }
            }
            n145 = property on="Motor" class="Clust (strict)"("Visible"=TRUE) -> ()  [unwired: 2 in, 2 out]
            n146 = property on="Value" class="Slide (strict)"("Value"=w258, "Scale.Minimum"=w260, "Scale.Maximum"=w259, "Scale.Increment"=w257) -> ()  [unwired: 2 in, 2 out]
            n147 = property on="On/Off" class="Bool (strict)"("Visible"=w262) -> ()  [unwired: 2 in, 2 out]
            n148 = property on="Test Slider" class="Slide (strict)"("Visible"=w262) -> ()  [unwired: 2 in, 2 out]
            n149 = property on="Test Ring" class="Ring (strict)"("Visible"=w262) -> ()  [unwired: 2 in, 2 out]
            n150 = property on="Rev/Fwd" class="Clust (strict)"("Visible"=w262) -> ()  [unwired: 2 in, 2 out]
          }
          frame "Servo" {
            w278 = FALSE ("Visible")
            n151 = call <vilib>:"NT Read Number.vi"("Name"=w280) -> ("Numeric"=w279:dbl)  [unwired: 9 in, 1 out]
            n152 = property on="Test Slider" class="Slide (strict)"("Visible"=TRUE, "Scale.Maximum"=170.0 ("Scale.Range:Maximum")) -> ()  [unwired: 2 in, 2 out]
            n153 = local write "Test Slider"(w279) -> ()
            n154 = property on="Motor" class="Clust (strict)"("Visible"=w278) -> ()  [unwired: 2 in, 2 out]
            n155 = property on="Rev/Fwd" class="Clust (strict)"("Visible"=w278) -> ()  [unwired: 2 in, 2 out]
            n156 = property on="On/Off" class="Bool (strict)"("Visible"=w278) -> ()  [unwired: 2 in, 2 out]
            n157 = property on="Test Ring" class="Ring (strict)"("Visible"=w278) -> ()  [unwired: 2 in, 2 out]
          }
          frame "Relay", "Solenoid" {
            w281 = FALSE ("Visible")
            n158 = property on="Motor" class="Clust (strict)"("Visible"=w281) -> ()  [unwired: 2 in, 2 out]
            n159 = property on="Test Slider" class="Slide (strict)"("Visible"=w281) -> ()  [unwired: 2 in, 2 out]
            n160 = Search and Replace String(input string=w282, search string="/Value  **", replace string="/Direction") -> (result string=w288:string)  [unwired: 5 in, 3 out]
            n161 = property on="Test Ring" class="Ring (strict)"("Visible"=w281) -> ()  [unwired: 2 in, 2 out]
            n162 = call <vilib>:"NT Read String.vi"("Name"=w288) -> ("String"=w286:string)  [unwired: 9 in, 1 out]
            n163 = Equal?(x="Both directions", y=w286) -> (x = y?=w284:bool)
            n164 = Not(x=w284) -> (.not. x?=w285:bool)
            n165 = property on="Rev/Fwd" class="Clust (strict)"("Visible"=w284) -> ()  [unwired: 2 in, 2 out]
            n166 = property on="On/Off" class="Bool (strict)"("Visible"=w285, "Caption.Text"=w283) -> ()  [unwired: 2 in, 2 out]
          }
          frame "Compressor", "Digital Out" {
            w291 = FALSE ("Visible")
            # "Get direction and finish"
            n167 = property on="Motor" class="Clust (strict)"("Visible"=w291) -> ()  [unwired: 2 in, 2 out]
            n168 = property on="Test Slider" class="Slide (strict)"("Visible"=w291) -> ()  [unwired: 2 in, 2 out]
            n169 = property on="Test Ring" class="Ring (strict)"("Visible"=w291) -> ()  [unwired: 2 in, 2 out]
            n170 = property on="On/Off" class="Bool (strict)"("Visible"=TRUE, "Caption.Text"=w292) -> ()  [unwired: 2 in, 2 out]
            n171 = property on="Rev/Fwd" class="Clust (strict)"("Visible"=FALSE) -> ()  [unwired: 2 in, 2 out]
          }
          frame "Camera" {
            n172 = call <vilib>:"Get Last Path Segment.vi"("String in"=w299) -> ("String out"=w300:string)  [unwired: 10 in]
            n173 = property on="On/Off" class="Bool (strict)"("Visible"=FALSE) -> ()  [unwired: 2 in, 2 out]
            n174 = property on="Motor" class="Clust (strict)"("Visible"=FALSE) -> ()  [unwired: 2 in, 2 out]
            n175 = property on="Rev/Fwd" class="Clust (strict)"("Visible"=FALSE) -> ()  [unwired: 2 in, 2 out]
            n176 = case shown="\"White Balance  **\"" w300 {
              tunnel: w299 -> [w306 w315 w324 w333 w342 _ w348]
              tunnel: w298 -> [w304 w312 w321 w330 w339 _ _]
              frame "Size  **" {
                n177 = Index Array(array=w304) -> (element=w303:cluster{string[]})  [unwired: 1 in]
                n178 = call <vilib>:"NT Read String.vi"("Name"=w306) -> ("String"=w305:string)  [unwired: 9 in, 1 out]
                n179 = Unbundle(w303) -> (w301:string[])
                n180 = Match First String(2:w301, 3:w305) -> (0:w302:i32)  [unwired: 1 out]
                n181 = property on="Test Ring" class="Ring (strict)"("Value"=w302, "Strings []"=w301) -> ()  [unwired: 2 in, 2 out]
                n182 = property on="Test Ring" class="Ring (strict)"("Visible"=TRUE) -> ()  [unwired: 2 in, 2 out]
                n183 = property on="Test Slider" class="Slide (strict)"("Visible"=FALSE) -> ()  [unwired: 2 in, 2 out]
              }
              frame "White Balance  **" {
                n184 = Index Array(array=w312, index=1) -> (element=w313:cluster{string[]})
                n185 = call <vilib>:"NT Read String.vi"("Name"=w315) -> ("String"=w314:string)  [unwired: 9 in, 1 out]
                n186 = Unbundle(w313) -> (w310:string[])
                n187 = Match First String(2:w310, 3:w314) -> (0:w309:i32)  [unwired: 1 out]
                n188 = property on="Test Ring" class="Ring (strict)"("Value"=w309, "Strings []"=w310) -> ()  [unwired: 2 in, 2 out]
                n189 = property on="Test Ring" class="Ring (strict)"("Visible"=TRUE) -> ()  [unwired: 2 in, 2 out]
                n190 = property on="Test Slider" class="Slide (strict)"("Visible"=FALSE) -> ()  [unwired: 2 in, 2 out]
              }
              frame "Exposure  **" {
                n191 = Index Array(array=w321, index=2) -> (element=w322:cluster{string[]})
                n192 = call <vilib>:"NT Read String.vi"("Name"=w324) -> ("String"=w323:string)  [unwired: 9 in, 1 out]
                n193 = Unbundle(w322) -> (w318:string[])
                n194 = Match First String(2:w318, 3:w323) -> (0:w319:i32)  [unwired: 1 out]
                n195 = property on="Test Ring" class="Ring (strict)"("Value"=w319, "Strings []"=w318) -> ()  [unwired: 2 in, 2 out]
                n196 = property on="Test Ring" class="Ring (strict)"("Visible"=TRUE) -> ()  [unwired: 2 in, 2 out]
                n197 = property on="Test Slider" class="Slide (strict)"("Visible"=FALSE) -> ()  [unwired: 2 in, 2 out]
              }
              frame "Exposure Priority  **" {
                n198 = Index Array(array=w330, index=3) -> (element=w331:cluster{string[]})
                n199 = call <vilib>:"NT Read String.vi"("Name"=w333) -> ("String"=w332:string)  [unwired: 9 in, 1 out]
                n200 = Unbundle(w331) -> (w327:string[])
                n201 = Match First String(2:w327, 3:w332) -> (0:w328:i32)  [unwired: 1 out]
                n202 = property on="Test Ring" class="Ring (strict)"("Value"=w328, "Strings []"=w327) -> ()  [unwired: 2 in, 2 out]
                n203 = property on="Test Ring" class="Ring (strict)"("Visible"=TRUE) -> ()  [unwired: 2 in, 2 out]
                n204 = property on="Test Slider" class="Slide (strict)"("Visible"=FALSE) -> ()  [unwired: 2 in, 2 out]
              }
              frame "Color Enable  **" {
                n205 = Index Array(array=w339, index=4) -> (element=w340:cluster{string[]})
                n206 = call <vilib>:"NT Read String.vi"("Name"=w342) -> ("String"=w341:string)  [unwired: 9 in, 1 out]
                n207 = Unbundle(w340) -> (w336:string[])
                n208 = Match First String(2:w336, 3:w341) -> (0:w337:i32)  [unwired: 1 out]
                n209 = property on="Test Ring" class="Ring (strict)"("Value"=w337, "Strings []"=w336) -> ()  [unwired: 2 in, 2 out]
                n210 = property on="Test Ring" class="Ring (strict)"("Visible"=TRUE) -> ()  [unwired: 2 in, 2 out]
                n211 = property on="Test Slider" class="Slide (strict)"("Visible"=FALSE) -> ()  [unwired: 2 in, 2 out]
              }
              frame Default {
                n212 = property on="Test Ring" class="Ring (strict)"("Visible"=FALSE) -> ()  [unwired: 2 in, 2 out]
                n213 = property on="Test Slider" class="Slide (strict)"("Visible"=FALSE) -> ()  [unwired: 2 in, 2 out]
              }
              frame "Brightness  **", "Color Level  **", "Compression  **", "FPS  **", "Sharpness  **" {
                n214 = call <vilib>:"NT Read Number.vi"("Name"=w348) -> ("Numeric"=w347:dbl)  [unwired: 9 in, 1 out]
                n215 = local write "Test Slider"(w347) -> ()
                n216 = property on="Test Slider" class="Slide (strict)"("Visible"=TRUE, "Scale.Maximum"=100.0 ("Scale.Range:Maximum")) -> ()  [unwired: 2 in, 2 out]
                n217 = property on="Test Ring" class="Ring (strict)"("Visible"=FALSE) -> ()  [unwired: 2 in, 2 out]
              }
            }
          }
        }
        n218 = property on="Progress" class="Clust (strict)"("Visible"=FALSE) -> ()  [unwired: 2 in, 2 out]
      }
      event "Test Name": Mouse Enter {
        # "Populate the ring with the list of tests"
        n219 = event-data() -> ()  [unwired: 1 in, 1 out]
        n220 = call <vilib>:"NT Read String Array.vi"("Name"="TestMode/TestList") -> ("String Array"=w356:string[])  [unwired: 9 in, 1 out]
        n221 = Build Array (concatenate)("Select the test to run...", w356) -> (w355:string[])
        n222 = property on="Test Name" class="Ring (strict)"("Strings []"=w355) -> ()  [unwired: 2 in, 2 out]
      }
      event "Test Name": Value Change {
        w358 = FALSE ("Visible")
        # "Tell the robot the test name to run"
        n223 = event-data() -> ("NewVal"=w362:u16)  [unwired: 1 in]
        n224 = property on="Test Name" class="Ring (strict)"() -> ("Strings []"=w363:string[])  [unwired: 2 in, 2 out]
        n225 = local write "Progress"(T6 {"Test Progress"=0, "Test Progress Text"=""} ("Progress")) -> ()
        n226 = Index Array(array=w363, index=w362) -> (element=w361:string)
        n227 = call <vilib>:"NT Write String.vi"("String"=w361, "Name"="TestMode/TestName") -> ()  [unwired: 9 in, 1 out]
        n228 = property on="Progress" class="Clust (strict)"("Visible"=TRUE) -> ()  [unwired: 2 in, 2 out]
        n229 = property on="Motor" class="Clust (strict)"("Visible"=w358) -> ()  [unwired: 2 in, 2 out]
        n230 = property on="Test Slider" class="Slide (strict)"("Visible"=w358) -> ()  [unwired: 2 in, 2 out]
        n231 = property on="On/Off" class="Bool (strict)"("Visible"=w358) -> ()  [unwired: 2 in, 2 out]
        n232 = property on="Rev/Fwd" class="Clust (strict)"("Visible"=w358) -> ()  [unwired: 2 in, 2 out]
        n233 = property on="Test Ring" class="Ring (strict)"("Visible"=w358) -> ()  [unwired: 2 in, 2 out]
      }
      event "Select Auto": Mouse Enter {
        # "Populate the combo box with the list of autonomous options"
        n234 = event-data() -> ()  [unwired: 1 in, 1 out]
        n235 = call <vilib>:"NT Read String Array.vi"("Name"="Auto List") -> ("String Array"=w365:string[])  [unwired: 9 in, 1 out]
        n236 = property on="Select Auto" class="CmbBox"("Strings[]"=w365) -> ()  [unwired: 2 in, 2 out]
      }
      event "Select Auto": Value Change {
        # "User modified the Auto Selection. Write to NT variable so robot knows."
        n237 = event-data() -> ("NewVal"=w368:string)  [unwired: 1 in]
        n238 = call <vilib>:"NT Write String.vi"("String"=w368, "Name"="Auto Selector") -> ()  [unwired: 9 in, 1 out]
      }
      event "Command Selection": Value Change {
        # "Get the params and show in table"
        n239 = event-data() -> ("NewVal"=w374:i32)  [unwired: 1 in]
        n240 = property on="Command Selection" class="MCListbox (strict)"() -> ("ItemNames"=w372:string[][])  [unwired: 2 in, 2 out]
        n241 = call <vilib>:"WPI_DashboardUpdate Command Params.vi"("NewVal"=w374, "Commands"=w372, "Param Tbl"=w373) -> ()  [unwired: 8 in, 1 out]
      }
      event "Execute Command": Value Change {
        # "Started one, Unique ID holds\nresponse"
        n242 = event-data() -> ()  [unwired: 1 in, 1 out]
        n243 = property on="Command Selection" class="MCListbox (strict)"() -> ("ItemNames"=w385:string[][])  [unwired: 2 in, 2 out]
        n244 = Index Array(array=w385, index (row)="Command Selection", index (col)=0) -> (element=w383:string)
        n245 = call <vilib>:"Invoke Commands.vi"("Command Params"="Command Params", "Function Name"=w383) -> ("Params"=w379:u8, "Started"=w378:bool)  [unwired: 7 in, 1 out]
        n246 = Array Subset(array="Command Params", length (row)=w379) -> (w380:string[][])  [unwired: 3 in]
        n247 = Select(t="Executing" ("Cmd Status"), s=w378, f="" ("Cmd Status")) -> (s? t:f=→"Cmd Status":string)
      }
      event "Command Selection": Double Click {
        n248 = event-data() -> ("Row"=w393:i32)  [unwired: 1 in]
        n249 = property on="Command Selection" class="MCListbox (strict)"() -> ("ItemNames"=w396:string[][])  [unwired: 2 in, 2 out]
        n250 = local read "Command Params"() -> (w392:string[][])
        n251 = Index Array(array=w396, index (row)=w393, index (col)=0) -> (element=w394:string)
        n252 = call <vilib>:"Invoke Commands.vi"("Command Params"=w392, "Function Name"=w394) -> ("Params"=w391:u8, "Started"=w386:bool)  [unwired: 7 in, 1 out]
        n253 = Array Subset(array=w392, length (row)=w391) -> (w390:string[][])  [unwired: 3 in]
        n254 = Select(t="Executing" ("Cmd Status"), s=w386, f="" ("Cmd Status")) -> (s? t:f=w387:string)
        n255 = local write "Cmd Status"(w387) -> ()
      }
      event "CheckList": Double Click {
        # "Shift clears all"
        # "Update symbols on the listbox"
        n256 = event-data() -> ("PlatMods.Shift"=w398:bool, "Row"=w400:i32)  [unwired: 1 in]
        n257 = case shown="True" w398 {
          tunnel: w400 -> [w404 _]
          tunnel: 1 -> [w403 _]
          frame False {
            n258 = property on="CheckList" class="LstBox (strict)"() -> ("Item Symbols"=w402:i32[])  [unwired: 2 in, 2 out]
            n259 = Replace Array Subset(array=w402, new element=w403, index=w404) -> (w401:i32[])
            n260 = property on="CheckList" class="LstBox (strict)"("Item Symbols"=w401) -> ()  [unwired: 2 in, 2 out]
          }
          frame True {
            w405 = 0 ("Top Row")
            n261 = property on="CheckList" class="LstBox (strict)"() -> ("Number of Rows"=w407:u32)  [unwired: 2 in, 2 out]
            n262 = Initialize Array(0, w407) -> (w406:i32[])
            n263 = property on="CheckList" class="LstBox (strict)"("Top Row"=w405, "Value"=w405, "Item Symbols"=w406) -> ()  [unwired: 2 in, 2 out]
          }
        }
      }
      event "CheckList": Key Down {
        # "Update symbols on the listbox\nLeft and right keys check and uncheck"
        n264 = event-data() -> ("VKey"=w411:T24)  [unwired: 1 in]
        n265 = case shown="\"Left\", \"Right\"" w411 {
          selector: w411 -> [w416 _]
          tunnel: eventvkey."Left" ("VKey") -> [w414 _]
          frame "Left", "Right" {
            n266 = Equal?(x=w414, y=w416) -> (x = y?=w415:bool)
            n267 = Select(t=0, s=w415, f=1) -> (s? t:f=w417:i32)
            n268 = property on="CheckList" class="LstBox (strict)"() -> ("Item Symbols"=w420:i32[])  [unwired: 2 in, 2 out]
            n269 = Replace Array Subset(array=w420, new element=w417, index="CheckList") -> (w419:i32[])
            n270 = property on="CheckList" class="LstBox (strict)"("Item Symbols"=w419) -> ()  [unwired: 2 in, 2 out]
          }
          frame Default {
          }
        }
      }
      event "Motor.Enable": Value Change {
        # "When the test mode otor enable helper is set, update that\ntree row item's value"
        n271 = event-data() -> ("NewVal"=w426:bool)  [unwired: 1 in]
        n272 = Unbundle("Motor") -> ("Value"=w425:dbl)  [unwired: 1 out]
        n273 = Select(t=w425, s=w426, f=0.0) -> (s? t:f=w423:dbl)
        n274 = call <vilib>:"NT Write Number.vi"("Numeric"=w423, "Name"=w422) -> ()  [unwired: 9 in, 1 out]
      }
      event "Test Slider": Value Change {
        # "When the test mode slider helper is set, update that\ntree row item's value"
        n275 = event-data() -> ("NewVal"=w429:dbl)  [unwired: 1 in]
        n276 = call <vilib>:"NT Write Number.vi"("Numeric"=w429, "Name"=w430) -> ()  [unwired: 9 in, 1 out]
      }
      event "On/Off": Value Change {
        # "When the test mode on/off helper value is set, update that\ntree row item's value"
        n277 = event-data() -> ("NewVal"=w434:bool)  [unwired: 1 in]
        n278 = Boolean To (0,1)(Boolean=w434) -> (0, 1=w433:i16)
        n279 = call <vilib>:"NT Write Number.vi"("Numeric"=w433, "Name"=w432) -> ()  [unwired: 9 in, 1 out]
      }
      event "Rev/Fwd": Value Change {
        # "When the test mode helper value for relays is set, update that\ntree row item's value"
        n280 = event-data() -> ("NewVal.Forward"=w442:bool, "NewVal.Reverse"=w441:bool)  [unwired: 1 in]
        n281 = Boolean To (0,1)(Boolean=w442) -> (0, 1=w438:i16)
        n282 = Boolean To (0,1)(Boolean=w441) -> (0, 1=w440:i16)
        n283 = Negate(x=w440) -> (-x=w439:i16)
        n284 = Add(x=w438, y=w439) -> (x+y=w437:i16)
        n285 = call <vilib>:"NT Write Number.vi"("Numeric"=w437, "Name"=w436) -> ()  [unwired: 9 in, 1 out]
      }
      event "Test Ring": Value Change {
        # "When a test mode helper value is selected from the ring,\nset the tree item's variable to the string value"
        n286 = event-data() -> ("NewVal"=w446:u16)  [unwired: 1 in]
        n287 = property on="Test Ring" class="Ring (strict)"() -> ("Strings []"=w447:string[])  [unwired: 2 in, 2 out]
        n288 = Index Array(array=w447, index=w446) -> (element=w445:string)
        n289 = call <vilib>:"NT Write String.vi"("String"=w445, "Name"=w444) -> ()  [unwired: 9 in, 1 out]
      }
      event "Rec Mode": Value Change {
        # "Update globals for recording mode and path to read log from.\nClear when logging and let NetworkTables set path for vision to\nuse."
        n290 = event-data() -> ("NewVal"=w458:enum32{"Stop", "Record", "Playback"})  [unwired: 1 in]
        n291 = global write "WPI_DashboardLogging Global.vi" "Logging Filename"(path "") -> ()
        n292 = global write "WPI_DashboardLogging Global.vi" "Recording"(w458) -> ()
        n293 = case shown="\"Playback\"" w458 {
          tunnel: w457 -> [_ w460 w469]
          tunnel: [_ _ w468] -> w455
          tunnel: [_ _ w467] -> _
          tunnel: w453 -> [_ _ w465]
          tunnel: cluster{i32, i32} {-250, 170} -> [_ _ w464]
          tunnel: [_ _ T25 {"Image Size"=TRUE, "Image Type"=TRUE, "Pixel Value"=TRUE, "ROI Information"=TRUE, "Zoom Factor"=FALSE} ("Image Information Shown:All Elements")] -> w448
          tunnel: [_ _ TRUE ("Zoom Factor")] -> w449
          tunnel: w451 -> [_ _ w461]
          frame Default {
          }
          frame "Stop", "Record" {
            # "Place Window too"
            n294 = invoke class="VI" method="FP.Close"(reference=w460) -> (reference out=w459:refnum<vi>)  [unwired: 2 in, 2 out]
            n295 = invoke class="VI" method="Abort VI"(reference=w459) -> ()  [unwired: 2 in, 3 out]
          }
          frame "Playback" {
            n296 = call "Open Playback Panel.vi"("Offset"=w464, "DB VI Ref"=w465, "Playback in"=w469) -> ("Playback out"=w466:refnum<vi>)  [unwired: 8 in]
            n297 = register-events(w466, w461) -> (reference out=w468:refnum<event-registration>, error out=w467:errorcluster)  [unwired: 2 in]
          }
        }
        n298 = property on="Camera Image Right" class="ImageControl"("Image Information Shown"=w448, "Image Information Visible"=w449) -> ()  [unwired: 2 in, 2 out]
        n299 = property on="Camera Image" class="ImageControl"("Image Information Shown"=w448, "Image Information Visible"=w449) -> ()  [unwired: 2 in, 2 out]
        n300 = call <vilib>:"WPI_DashboardNT Log FieldName Cache.vi"("Operation"=enum16{"Lookup/Add", "Index", "Clear"}."Clear") -> ()  [unwired: 8 in, 3 out]
      }
      event Panel Close {
        w471 = enum32{"Stop", "Record", "Playback"}."Stop" ("Rec Mode")
        # "Playback window has been closed, abort"
        n301 = event-data() -> ()  [unwired: 1 in, 4 out]
        n302 = local write "Rec Mode"(w471) -> ()
        n303 = global write "WPI_DashboardLogging Global.vi" "Recording"(w471) -> ()
      }
      event Panel Close {
        # "Abort playback window and ourself"
        n304 = event-data() -> ()  [unwired: 1 in, 4 out]
        n305 = invoke class="VI" method="FP.Close"(reference=w475) -> (reference out=w474:refnum<vi>)  [unwired: 2 in, 2 out]
        n306 = invoke class="VI" method="Abort VI"(reference=w474) -> (error out=w473:errorcluster)  [unwired: 2 in, 2 out]
        n307 = invoke class="VI" method="Abort VI"(error in=w473) -> ()  [unwired: 2 in, 3 out]
      }
      event User Event {
        n308 = event-data() -> ("IDs"=w482:cluster{"RPC field ID":u16, "Unique ID":u16}, "String"=w481:string)  [unwired: 1 in]
        n309 = Bundle("IDs"=w482, "String"=w481) -> (w480:T9)  [unwired: 1 in]
        n310 = call <vilib>:"Retrieve RPC Response.vi"("RPC Response"=w480) -> ("Output"=w478:string[][])  [unwired: 10 in]
        n311 = Build Array (concatenate)(w476, w478) -> (w477:string[][])
        n312 = local write "Command Params"(w477) -> ()
        n313 = local write "Cmd Status"("" ("Cmd Status")) -> ()
      }
      event "Tree": Double Click {
        n314 = event-data() -> ("PlatMods"=w488:T28, "Tag"=w485:string)  [unwired: 1 in]
        n315 = Unbundle(w488) -> ("Shift"=w487:bool)  [unwired: 4 out]
        n316 = String Subset(string=w485, length (rest)=1 ("length (rest)")) -> (substring=w484:string)  [unwired: 1 in]
        n317 = Not(x=w487) -> (.not. x?=w486:bool)
        n318 = case shown="\"/\"" w484 {
          tunnel: w485 -> [_ w491]
          tunnel: w486 -> [_ w490]
          frame Default {
          }
          frame "/" {
            n319 = call <vilib>:"NT Update Persistence.vi"("Persistence"=w490, "Name"=w491) -> ()  [unwired: 9 in, 1 out]
          }
        }
      }
    }
  }
  n320 = while {
    tunnel: w69 -> [w493]
    i -> [w496]
    stop <- FALSE stop-if-true
    n321 = Wait (ms)(milliseconds to wait=u32 100) -> ()  [unwired: 1 out]
    n322 = case shown="\"Playback\"" "Rec Mode" {
      tunnel: w496 -> [_ _ w511]
      tunnel: [u32 2829099 ("Base Color") u32 11141120 ("Target Color") w500] -> w492
      frame "Stop", Default {
        # "Reset the color, extra updates don't cost much"
      }
      frame "Record" {
      }
      frame "Playback" {
        # "Playback"
        n323 = Quotient & Remainder(x=w511, y=u32 50 ("milliseconds to wait")) -> (x-y*floor(x/y)=w507:u32)  [unwired: 1 out]
        n324 = Divide(x=w507, y=u32 50 ("milliseconds to wait")) -> (x/y=w504:dbl)
        n325 = Multiply(x=6.283185307179586, y=w504) -> (x*y=w509:dbl)
        n326 = Sine(x=w509) -> (sin(x)=w508:dbl)
        n327 = Absolute Value(x=w508) -> (abs(x)=w501:dbl)
        n328 = call "Interpolate RGB Color.vi"("Proportion"=w501, "Target Color"=u32 30976, "Base Color"=u32 2829099) -> ("Result Color"=w500:u32)  [unwired: 8 in]
      }
    }
    n329 = property class="Pane"(reference=w493, "PaneColor"=w492) -> ()  [unwired: 1 in, 2 out]
  }
  n330 = local write "Dashboard Tab"(T2."Drive" ("Dashboard Tab")) -> ()
  n331 = property on="On/Off" class="Bool (strict)"("Visible"=w40) -> ()  [unwired: 2 in, 2 out]
  n332 = property on="Motor" class="Clust (strict)"("Visible"=w40) -> ()  [unwired: 2 in, 2 out]
  n333 = property on="Progress" class="Clust (strict)"("Visible"=w40) -> ()  [unwired: 2 in, 2 out]
  n334 = property on="Test Ring" class="Ring (strict)"("Visible"=w40) -> ()  [unwired: 2 in, 2 out]
  n335 = property on="Rev/Fwd" class="Clust (strict)"("Visible"=w40) -> ()  [unwired: 2 in, 2 out]
  n336 = while {
    tunnel: u16 1741 ("timeout ms (25000)") -> [w513]
    stop <- FALSE stop-if-true
    n337 = TCP Create Listener(10:w513) -> (0:w512:errorcluster, 3:w514:refnum<k5>)  [unwired: 4 in, 1 out]
    n338 = case shown="No Error" w512 {
      selector: w512 -> [w516 _]
      tunnel: w514 -> [w517 _]
      frame No Error {
        n339 = while {
          tunnel: w517 -> [w520]
          tunnel: w516 -> [w519]
          stop <- FALSE stop-if-true
          n340 = TCP Wait On Listener(8:w519, 11:w520) -> (0:w521:errorcluster, 4:w522:refnum<k5>)  [unwired: 2 in, 3 out]
          n341 = local write "TCP"(w522) -> ()
          n342 = case shown="No Error" w521 {
            frame No Error {
            }
            frame Error {
              n343 = Wait (ms)(milliseconds to wait=u32 1000) -> ()  [unwired: 1 out]
            }
          }
        }
      }
      frame Error {
        n344 = Wait (ms)(milliseconds to wait=u32 1000) -> ()  [unwired: 1 out]
      }
    }
  }
  n345 = local write "Command Selection"(u16 0 ("milliseconds to wait")) -> ()
  n346 = local write "Command Params"(string[][] [] ("Command Params")) -> ()
  n347 = global write "WPI_DashboardLogging Global.vi" "Recording"(w63) -> ()
  n348 = local write "Rec Mode"(w63) -> ()
  n349 = call <vilib>:"NT Write String.vi"("String"="Select Auto", "Name"="Auto Selector") -> ()  [unwired: 9 in, 1 out]
  n350 = call-poly <vilib>:"NT Read Value.vi"("Name"="Vision Toggle") -> ("Boolean"=w3:bool)  [unwired: 9 in, 1 out]
  n351 = case shown="True" w3 {
    tunnel: [1.0 ("Numeric") 0.0 ("Numeric")] -> w1
    frame False {
    }
    frame True {
    }
  }
  n352 = call-poly <vilib>:"NT Write Value.vi"("Numeric"=w1, "Name"="/limelight/camMode") -> ()  [unwired: 9 in, 1 out]
